vi "bug man P start.vi"() -> ()   [LabVIEW 2019]
doc: "This is the Main VI for the bug manual power controller.\n\nThe user can control the temp via manual power control at any time during operation. \n\nJuan Gamez\nP3600\nCSUSB Physics"
uses:
  components/typedefs/exp sequence.ctl
  components/typedefs/PID exec cluster.ctl
  components/typedefs/bug temp file info.ctl
  components/typedefs/temp mode enum.ctl
  components/globals/Bug man temp globals.vi
panel:
  out "Power":dbl format="%#_4g"
  out "Temp":dbl
  out "Temperature Graph":cluster{"t hist":dbl[], "T hist":dbl[]}[](graph)=[{"t hist"=[0.681, 1.01, 1.338, 1.667, 1.996, 2.323, 2.651, 2.979, 3.308, 3.636, 3.966, 4.294, 4.622, 4.95, 5.282, 5.614, 5.949, 6.292, 6.624, 6.956, 7.29, 7.629, 7.962, 8.298, 8.632, 8.961, 9.305, 9.649, 9.982, 10.321], "T hist"=[28.221637848568264, 28.335463471473247, 28.45177291236797, 28.578054212374127, 28.712611988419383, 28.84616557500516, 28.98818760788282, 29.12927903863408, 29.273265947327218, 29.420201611602806, 29.566232905582694, 29.70936480151545, 29.857453821818012, 29.996629768200933, 30.14076143529155, 30.28185384495856, 30.41983725429435, 30.556691662116748, 30.68413877422978, 30.810295121327613, 30.930958632049965, 31.052323535552546, 31.161736118199713, 31.269603761681765, 31.37376795546072, 31.474170088455764, 31.568601926879808, 31.65482002616045, 31.741394285589706, 31.819617943507183]}, {"t hist"=[0.681, 1.01, 1.338, 1.667, 1.996, 2.323, 2.651, 2.979, 3.308, 3.636, 3.966, 4.294, 4.622, 4.95, 5.282, 5.614, 5.949, 6.292, 6.624, 6.956, 7.29, 7.629, 7.962, 8.298, 8.632, 8.961, 9.305, 9.649, 9.982, 10.321], "T hist"=[61.64927318018057, 60.87935633362467, 59.91081367089514, 59.07163506893572, 58.05431280608125, 56.97210065484677, 55.985935993807566, 54.81990049342825, 53.76683173570311, 52.62763554543207, 51.438400944419776, 50.316274027152325, 49.20160602426924, 47.947916986672055, 46.929584951781365, 45.70234026722682, 44.56571400351665, 43.46069894631547, 42.34612964276051, 41.30873367322221, 40.22693480489379, 39.23489588337625, 38.167150974118684, 37.28797871837572, 36.32680632996466, 35.39340435832317, 34.47125846281813, 33.68091084957889, 32.922923294982894, 32.02199191964152]}]
  out "exit loc":bool
  out "Exp Seq":T1 caption="Experimental Sequence"
  in  "proceed":bool
  in  "exit":bool
  in  "exit":bool
  out "Total elapsed time (s)":i32=10
  in  "Manual Power":dbl(slide) scale=0.0..1.0
  out "meas index":i32
  # "Bug Experiment \nManual Temperature Control"
  # "Note: This TAB is under system control, \nthe others are under user control"
  # "Juan Gamez\nP3600\nCSUSB-Physics"
  # "Experiment Completed"
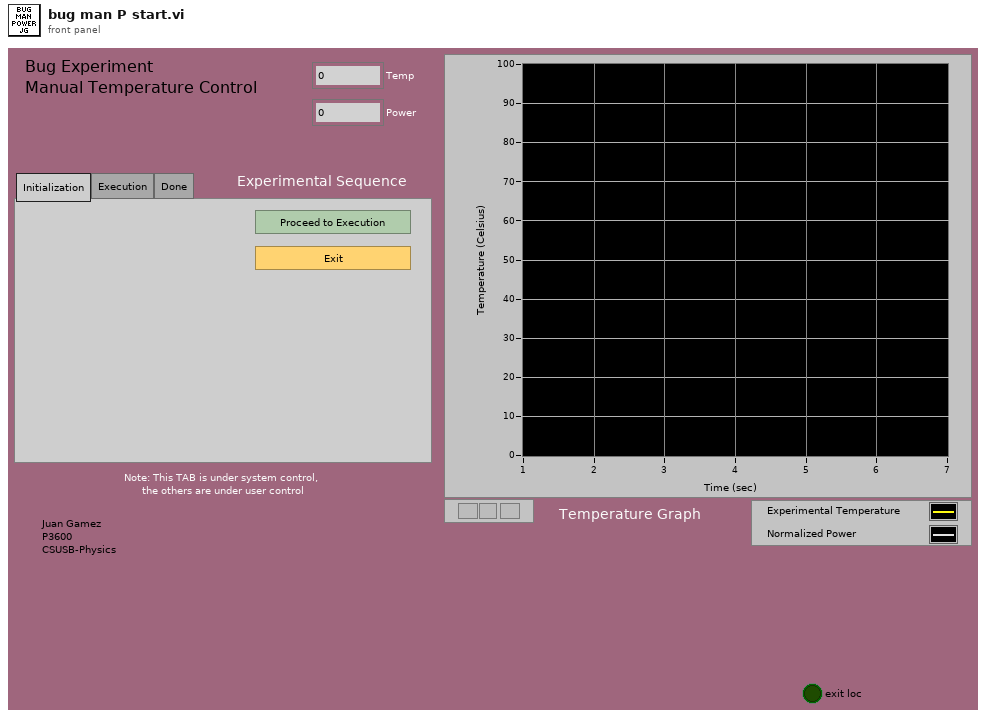
[diagram p1: front panel]
types:
  T1 = typedef "exp sequence.ctl" = enum32{"Initialization", "Execution", "Done"}
  T2 = typedef "temp mode enum.ctl" = enum16{"Setting up", "Listening to exec", "Exit"}
  T3 = typedef "PID exec cluster.ctl" = cluster{"T log file":T4, "error":errorcluster, "elapsed time (s)":dbl}
  T4 = typedef "bug temp file info.ctl" = cluster{"log exists":bool, "File refnum":refnum<file>, "temp log file path":path}
  T5 = typedef "temp cont cluster.ctl" = cluster{"exec":T6, "T status":T7, "utility":T8}
  T6 = typedef "temp exec cluster.ctl" = cluster{"T mode":T2, "man power":dbl, "log":bool}
  T7 = typedef "temp indicator.ctl" = cluster{"Temp":dbl, "Power":dbl}
  T8 = typedef "temp cont utility.ctl" = cluster{"meas index":i32, "wait (ms)":i32, "H Vmax":dbl, "power out":dbl, "heat volt out":dbl, "heat volt in":dbl, "therm volt":dbl, "t T P hist":dbl[][]}
  T9 = typedef "DAQ T state cluster.ctl" = cluster{"DAQ state":T10, "device":tag, "start (ms)":i32, "error":errorcluster, "T cont":T5}
  T10 = typedef "DAQ T state enum.ctl" = enum16{"Global comm", "Meas T & P", "Man Power set", "Output Power", "Wait", "Exit"}
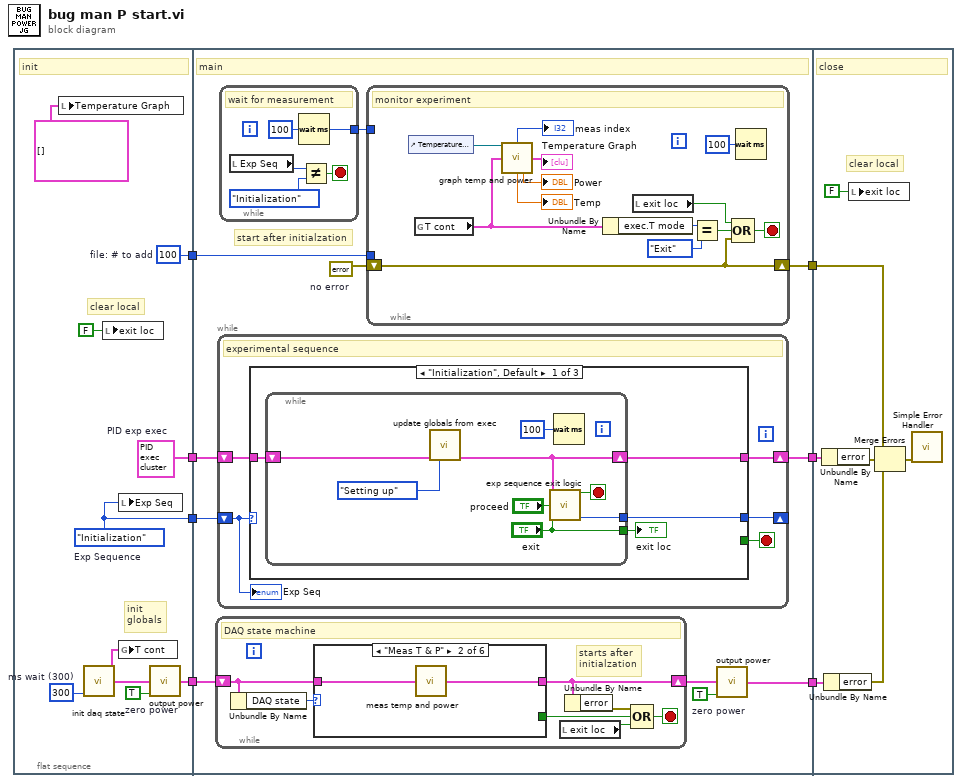
[diagram p0: block diagram]
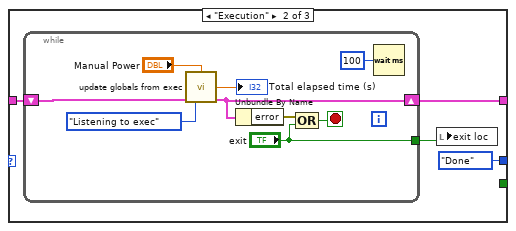
[diagram p2: hidden frame]
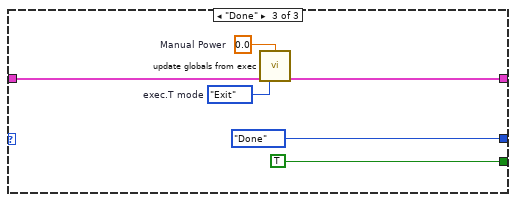
[diagram p3: hidden frame]
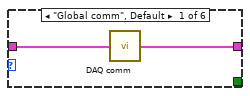
[diagram p4: hidden frame]
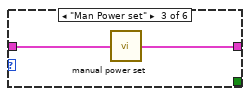
[diagram p5: hidden frame]
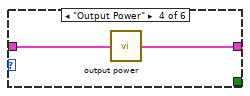
[diagram p6: hidden frame]
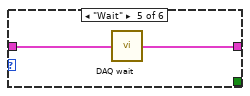
[diagram p7: hidden frame]
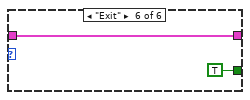
[diagram p8: hidden frame]
diagram:
  n1 = flat-sequence {
    tunnel: [w10] -> w4
    tunnel: [w16] -> w3
    tunnel: [w13] -> w2
    tunnel: [w8] -> w1
    tunnel: [w28] -> w7
    tunnel: [w27] -> w6
    tunnel: [w20] -> w5
    tunnel: w4 -> [w26]
    tunnel: w3 -> [w25]
    tunnel: w2 -> [w24]
    tunnel: w1 -> [w18]
    tunnel: w7 -> [w105]
    tunnel: w6 -> [w104]
    tunnel: w5 -> [w103]
    frame #0 {
      w8 = 100  # file: # to add
      w9 = TRUE  # zero power
      w16 = T3 {"T log file"={"log exists"=FALSE, "File refnum"=refnum, "temp log file path"=path ""}, "error"={"status"=FALSE, "code"=0, "source"=""}, "elapsed time (s)"=0.0}  # PID exp exec
      w13 = exp_sequence."Initialization"  # Exp Sequence
      w17 = 300  # ms wait (300)
      # "clear local"
      # "init\nglobals"
      # "init"
      n2 = local write "Temperature Graph"(cluster{"t hist":dbl[], "T hist":dbl[]}[] [] ("Temperature Graph")) -> ()
      n3 = call "init daq state.vi"("T cont wait time (ms)"=w17) -> ("T cont out for global update"=w12:T5, "DAQ state start out"=w11:T9)  [unwired: 13 in]
      n4 = local write "exit loc"(FALSE ("exit")) -> ()
      n5 = local write "Exp Seq"(w13) -> ()
      n6 = global write "Bug man temp globals.vi" "T cont"(w12) -> ()
      n7 = call "output power.vi"("DAQ state cluster in"=w11, "zero power"=w9) -> ("DAQ state cluster out"=w10:T9)  [unwired: 13 in]
    }
    frame #1 {
      w19 = errorcluster {"status"=FALSE, "code"=0, "source"=""}  # no error
      w22 = TRUE  # zero power
      # "start after initialzation"
      # "main"
      n8 = while {
        shift-right: [w84] -> w21
        shift-left: w26 -> [w85]
        stop <- w88 stop-if-true
        # "starts after \ninitialzation"
        # "DAQ state machine"
        n9 = Unbundle By Name(w85) -> ("DAQ state"=w86:T10)
        n10 = case shown="\"Meas T & P\"" w86 {
          tunnel: [_ _ _ _ _ TRUE] -> w87
          tunnel: w85 -> [w91 w93 w95 w97 w99 w100]
          tunnel: [w90 w92 w94 w96 w98 w100] -> w84
          frame "Global comm", Default {
            n11 = call "DAQ comm.vi"("DAQ T state cluster in"=w91) -> ("DAQ T state cluster out"=w90:T9)  [unwired: 14 in]
          }
          frame "Meas T & P" {
            n12 = call "meas temp and power.vi"("DAQ state cluster in"=w93) -> ("DAQ state cluster out"=w92:T9)  [unwired: 14 in]
          }
          frame "Man Power set" {
            n13 = call "manual power set.vi"("DAQ state cluster in"=w95) -> ("DAQ state cluster out"=w94:T9)  [unwired: 14 in]
          }
          frame "Output Power" {
            n14 = call "output power.vi"("DAQ state cluster in"=w97) -> ("DAQ state cluster out"=w96:T9)  [unwired: 14 in]
          }
          frame "Wait" {
            n15 = call "DAQ wait.vi"("DAQ state cluster in"=w99) -> ("DAQ state cluster out"=w98:T9)  [unwired: 14 in]
          }
          frame "Exit" {
          }
        }
        n16 = local read "exit loc"() -> (w83:bool)
        n17 = Unbundle By Name(w84) -> ("error"=w89:errorcluster)
        n18 = Compound Arithmetic op=OR(w89, w87, w83) -> (w88:bool)
      }
      n19 = while {
        shift-right: [w48] -> _
        shift-left: w24 -> [w49]
        shift-right: [w50] -> w28
        shift-left: w25 -> [w51]
        stop <- w47 stop-if-true
        # "experimental sequence"
        n20 = case shown="\"Initialization\", Default" w49 {
          tunnel: w51 -> [w54 w67 w80]
          tunnel: [w55 w66 w79] -> w50
          tunnel: [w53 exp_sequence."Done" ("Experimental Sequence") exp_sequence."Done" ("Experimental Sequence")] -> w48
          tunnel: [_ _ TRUE] -> w47
          frame "Initialization", Default {
            n21 = while {
              shift-right: [w58] -> w55
              shift-left: w54 -> [w56]
              tunnel: [w60] -> w53
              tunnel: ["exit"] -> w52
              stop <- w61 stop-if-true
              n22 = call "update globals from exec.vi"("PID exp exec"=w56, "exec.T mode"=temp_mode_enum."Setting up") -> ("PID exp exec out"=w58:T3)  [unwired: 12 in, 1 out]
              n23 = call "exp sequence exit logic.vi"("PID exp exec in"=w58, "proceed"="proceed", "exit"="exit") -> ("stop loop"=w61:bool, "Experimental Sequence"=w60:T1)  [unwired: 11 in]
              n24 = Wait (ms)(milliseconds to wait=u32 100) -> ()  [unwired: 1 out]
            }
            "exit loc" <- w52
          }
          frame "Execution" {
            n25 = while {
              shift-right: [w73] -> w66
              shift-left: w67 -> [w68]
              tunnel: ["exit"] -> w65
              stop <- w74 stop-if-true
              n26 = call "update globals from exec.vi"("Manual Power"="Manual Power", "PID exp exec"=w68, "exec.T mode"=temp_mode_enum."Listening to exec") -> ("Total elapsed time (s)"=→"Total elapsed time (s)":dbl, "PID exp exec out"=w73:T3)  [unwired: 11 in]
              n27 = Unbundle By Name(w73) -> ("error"=w75:errorcluster)
              n28 = Compound Arithmetic op=OR(w75, "exit") -> (w74:bool)
              n29 = Wait (ms)(milliseconds to wait=u32 100) -> ()  [unwired: 1 out]
            }
            n30 = local write "exit loc"(w65) -> ()
          }
          frame "Done" {
            w78 = 0.0  # Manual Power
            w77 = temp_mode_enum."Exit"  # exec.T mode
            n31 = call "update globals from exec.vi"("Manual Power"=w78, "PID exp exec"=w80, "exec.T mode"=w77) -> ("PID exp exec out"=w79:T3)  [unwired: 11 in, 1 out]
          }
        }
        "Exp Seq" <- w49
      }
      n32 = while {
        tunnel: [w29] -> w23
        stop <- w30 stop-if-true
        # "wait for measurement"
        n33 = local read "Exp Seq"() -> (w32:T1)
        n34 = Wait (ms)(milliseconds to wait=u32 100) -> (millisecond timer value=w29:u32)
        n35 = Not Equal?(x=w32, y=exp_sequence."Initialization" ("Experimental Sequence")) -> (x != y?=w30:bool)
      }
      n36 = while {
        shift-right: [w34] -> w27
        shift-left: w19 -> [w34]
        tunnel: w23 -> [_]
        tunnel: w18 -> [_]
        stop <- w43 stop-if-true
        # "monitor experiment"
        n37 = control-ref of="Temperature Graph"() -> (w37:refnum<vi>)
        n38 = global read "Bug man temp globals.vi" "T cont"() -> (w41:T5)
        n39 = call "graph temp and power.vi"("Temperature Graph"=w37, "T cont"=w41) -> ("meas index"=→"meas index":i32, "T and P graph"=→"Temperature Graph":cluster{"t hist":dbl[], "T hist":dbl[]}[], "T status.Temp"=→"Temp":dbl, "T status.Power"=→"Power":dbl)  [unwired: 10 in]
        n40 = Unbundle By Name(w41) -> ("exec.T mode"=w42:T2)
        n41 = local read "exit loc"() -> (w40:bool)
        n42 = Equal?(x=w42, y=temp_mode_enum."Exit" ("exec.T mode")) -> (x = y?=w44:bool)
        n43 = Compound Arithmetic op=OR(w40, w44, w34) -> (w43:bool)
        n44 = Wait (ms)(milliseconds to wait=u32 100) -> ()  [unwired: 1 out]
      }
      n45 = call "output power.vi"("DAQ state cluster in"=w21, "zero power"=w22) -> ("DAQ state cluster out"=w20:T9)  [unwired: 13 in]
    }
    frame #2 {
      # "clear local"
      # "close"
      n46 = Unbundle By Name(w105) -> ("error"=w108:errorcluster)
      n47 = Unbundle By Name(w103) -> ("error"=w107:errorcluster)
      n48 = local write "exit loc"(FALSE ("exit")) -> ()
      n49 = Merge Errors(w104, w108, w107) -> (w106:errorcluster)
      n50 = call <vilib>:"Simple Error Handler.vi"("error in (no error)"=w106) -> ()  [unwired: 4 in, 5 out]
    }
  }
